vi "Create ListImp_Empty.vi"(5 "ListImp_Empty in":refnum<class "ListImp_Empty.lvclass">, 8 "error in (no error)":errorcluster, 11 "ListImp":refnum<class "ListImp.lvclass">) -> (0 "error out":errorcluster, 3 "ListImp_Empty out":refnum<class "ListImp_Empty.lvclass">)   [LabVIEW 2013, in "ListImp_Empty.lvclass"]
uses:
  ListImp_Empty.lvclass
  source/LapDog.Collections.Lists/ListImp/ListImp.lvclass
  ListImp_Empty.lvclass/ListImp_Empty.ctl
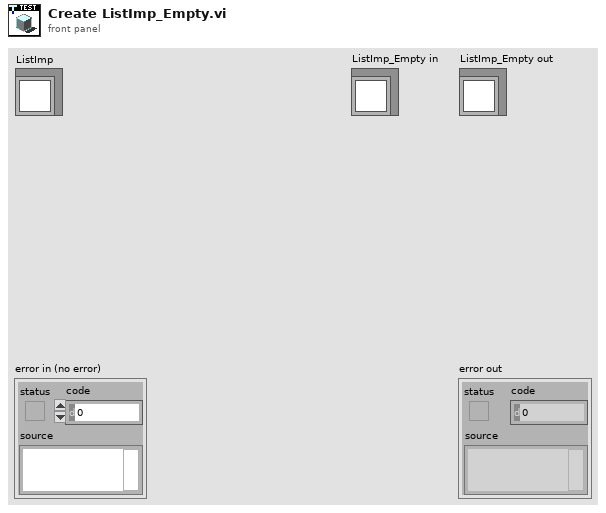
[diagram p1: front panel]
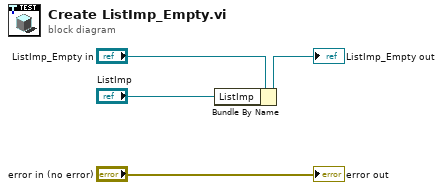
[diagram p0: block diagram]
diagram:
  n1 = Bundle By Name(cluster="ListImp_Empty in", "ListImp"="ListImp") -> (→"ListImp_Empty out":refnum<class "ListImp_Empty.lvclass">)
  "error out" <- "error in (no error)"
